vi "Connect.vi"   [LabVIEW 2020, in "NI_SFTP.lvlib"]
doc: "Connects to an SFTP server. The instance VI determines which SSH client to use."
uses:
  <vilib>/net/SFTP/NI_SFTP.lvlib
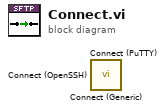
[diagram p0: block diagram]
diagram:
  n1 = call <vilib>:"Connect (Generic).vi"() -> ()  [unwired: 10 in, 2 out]
  n2 = call <vilib>:"Connect (PuTTY).vi"() -> ()  [unwired: 10 in, 2 out]
  n3 = call <vilib>:"Connect (OpenSSH).vi"() -> ()  [unwired: 10 in, 2 out]
